vi "Control Panel Values Changed.vi"(8 "error in (no error)":errorcluster, 9 "Old value":variant, 10 "New value":variant, 11 "Cryomagnetics Power Supply in":refnum<class "Cryomagnetics Power Supply.lvclass">) -> (0 "error out":errorcluster, 3 "Cryomagnetics Power Supply out":refnum<class "Cryomagnetics Power Supply.lvclass">)   [LabVIEW 2015, in "Cryomagnetics Power Supply.lvclass"]
uses:
  Cryomagnetics Power Supply.lvclass
  Cryomagnetics Control Panel Data.ctl
  Sweep mode.ctl
  Instrument/Read VISA Resource.vi
  Instrument/Write VISA Resource.vi
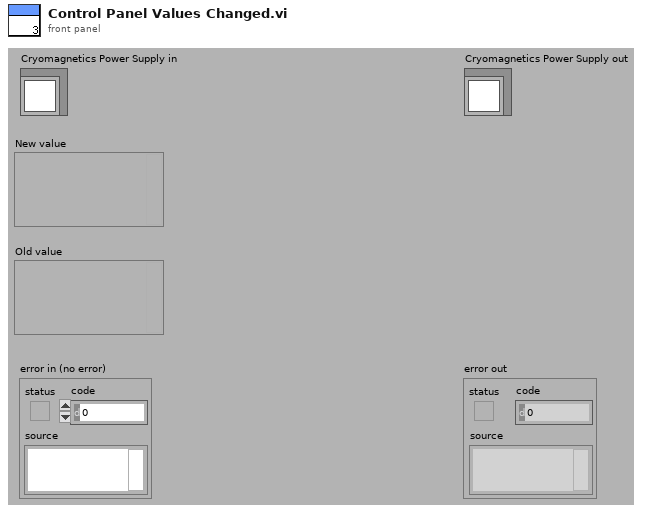
[diagram p1: front panel]
types:
  T1 = typedef "Cryomagnetics Control Panel Data.ctl" = cluster{"Persistent switch heater":bool, "Rates, A/s":dbl[], "Ranges, A":dbl[], "High limit, kG":dbl, "Low limit, kG":dbl, "Sweep ":T2, "Fast rate":dbl}
  T2 = typedef "Sweep mode.ctl" = cluster{"zero":bool, "sweep up":bool, "sweep down":bool, "fast sweep":bool}
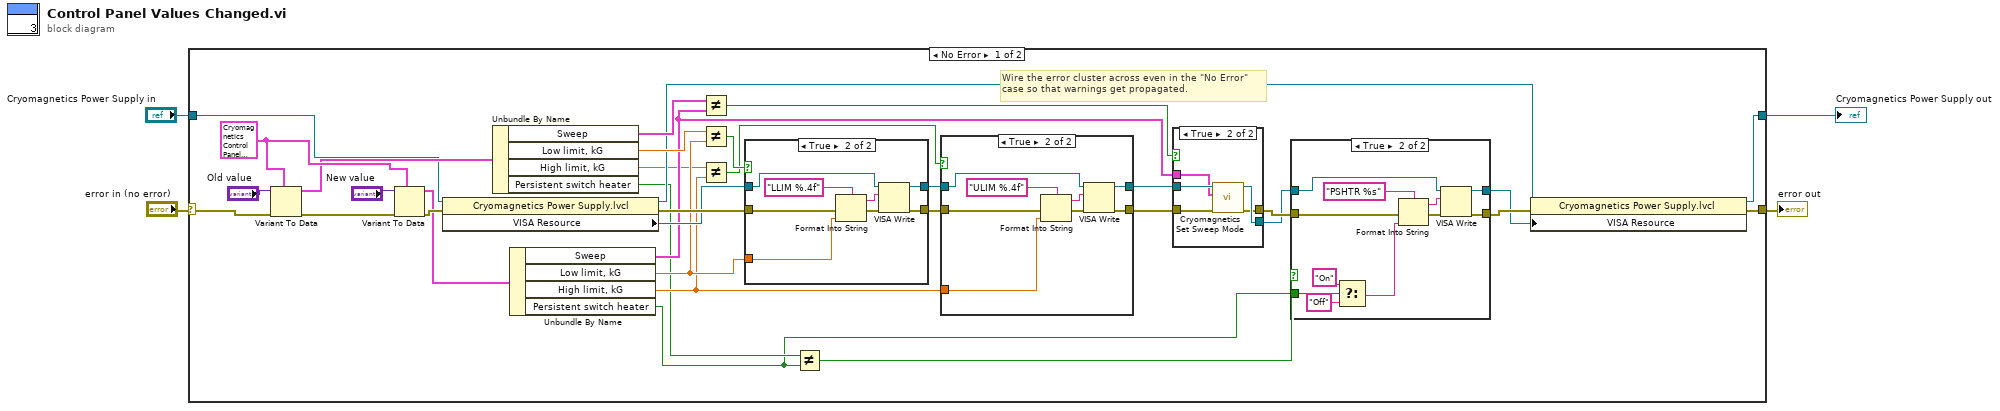
[diagram p0: block diagram]
diagram:
  n1 = case shown="No Error" "error in (no error)" {
    selector: "error in (no error)" -> [w21 w80]
    tunnel: [w20 w80] -> w3
    tunnel: [w19 w79] -> w1
    tunnel: "Cryomagnetics Power Supply in" -> [w22 w79]
    frame No Error {
      w34 = T1 {"Persistent switch heater"=FALSE, "Rates, A/s"=[0.01, 0.05, 0.0001, 0.0001, 0.0001], "Ranges, A"=[50.0, 76.9, 80.0, 85.0, 100.0], "High limit, kG"=0.01, "Low limit, kG"=0.0, "Sweep "={"zero"=FALSE, "sweep up"=FALSE, "sweep down"=FALSE, "fast sweep"=FALSE}, "Fast rate"=0.0} ("Data")
      # "Wire the error cluster across even in the \"No Error\"\ncase so that warnings get propagated."
      n2 = Variant To Data(error in=w21, type=w34, Variant="Old value") -> (data=w31:T1, error out=w38:errorcluster)
      n3 = Variant To Data(error in=w38, type=w34, Variant="New value") -> (data=w30:T1, error out=w37:errorcluster)
      n4 = property class="Cryomagnetics Power Supply.lvcl"(reference=w22, error in=w37) -> (reference out=w23:refnum<class "Cryomagnetics Power Supply.lvclass">, error out=w29:errorcluster, "VISA Resource"=w28:refnum<visa-resource-name>)
      n5 = Unbundle By Name(w31) -> ("Sweep"=w32:T2, "Low limit, kG"=w33:dbl, "High limit, kG"=w17:dbl, "Persistent switch heater"=w7:bool)
      n6 = Unbundle By Name(w30) -> ("Sweep"=w25:T2, "Low limit, kG"=w26:dbl, "High limit, kG"=w16:dbl, "Persistent switch heater"=w6:bool)
      n7 = Not Equal?(x=w32, y=w25) -> (x != y?=w24:bool)
      n8 = Not Equal?(x=w33, y=w26) -> (x != y?=w27:bool)
      n9 = Not Equal?(x=w17, y=w16) -> (x != y?=w18:bool)
      n10 = case shown="True" w27 {
        tunnel: w29 -> [w70 w78]
        tunnel: w28 -> [w69 w77]
        tunnel: w26 -> [_ w73]
        tunnel: [w70 w76] -> w12
        tunnel: [w69 w75] -> w15
        frame False {
        }
        frame True {
          n11 = Format Into String(format string="LLIM %.4f", error in=w78, w73) -> (resulting string=w71:string, error out=w74:errorcluster)  [unwired: 1 in]
          n12 = VISA Write(VISA resource name=w77, write buffer=w71, error in (no error)=w74) -> (VISA resource name out=w75:refnum<visa-resource-name>, error out=w76:errorcluster)  [unwired: 1 out]
        }
      }
      n13 = Not Equal?(x=w7, y=w6) -> (x != y?=w5:bool)
      n14 = case shown="True" w18 {
        tunnel: w12 -> [w53 w61]
        tunnel: w15 -> [w52 w60]
        tunnel: w16 -> [_ w56]
        tunnel: [w53 w59] -> w13
        tunnel: [w52 w58] -> w14
        frame False {
        }
        frame True {
          n15 = Format Into String(format string="ULIM %.4f", error in=w61, w56) -> (resulting string=w54:string, error out=w57:errorcluster)  [unwired: 1 in]
          n16 = VISA Write(VISA resource name=w60, write buffer=w54, error in (no error)=w57) -> (VISA resource name out=w58:refnum<visa-resource-name>, error out=w59:errorcluster)  [unwired: 1 out]
        }
      }
      n17 = case shown="True" w24 {
        tunnel: w13 -> [w63 w68]
        tunnel: w14 -> [w62 w67]
        tunnel: w25 -> [_ w64]
        tunnel: [w62 w66] -> w9
        tunnel: [w63 w65] -> w11
        frame False {
        }
        frame True {
          n18 = call "Cryomagnetics Set Sweep Mode.vi"("error in (no error)"=w68, "sweep mode"=w64, "VISA Resource Name"=w67) -> ("error out"=w65:errorcluster, "VISA Resource Name Out"=w66:refnum<visa-resource-name>)  [unwired: 7 in]
        }
      }
      n19 = case shown="True" w5 {
        tunnel: w11 -> [w40 w51]
        tunnel: w9 -> [w39 w50]
        tunnel: w6 -> [_ w46]
        tunnel: [w40 w49] -> w10
        tunnel: [w39 w48] -> w8
        frame False {
        }
        frame True {
          n20 = Select(t="On", s=w46, f="Off") -> (s? t:f=w43:string)
          n21 = Format Into String(format string="PSHTR %s", error in=w51, w43) -> (resulting string=w44:string, error out=w47:errorcluster)  [unwired: 1 in]
          n22 = VISA Write(VISA resource name=w50, write buffer=w44, error in (no error)=w47) -> (VISA resource name out=w48:refnum<visa-resource-name>, error out=w49:errorcluster)  [unwired: 1 out]
        }
      }
      n23 = property class="Cryomagnetics Power Supply.lvcl"(reference=w23, error in=w10, "VISA Resource"=w8) -> (reference out=w19:refnum<class "Cryomagnetics Power Supply.lvclass">, error out=w20:errorcluster)
    }
    frame Error {
    }
  }
  "error out" <- w3
  "Cryomagnetics Power Supply out" <- w1
